vi "Test Production Unit API.vi"() -> ()   [LabVIEW 2025]
doc: "My Module API Tester.\n_____\nBased on DQMH Dev Tools: Project Template 7.1.2.1547."
uses:
  Production Unit.lvlib
  <vilib>/Utility/error.llb/DialogType.ctl
panel:
  out "last error":errorcluster
  in  "Show Diagram on Init":bool
  in  "Run as Singleton?":bool
  in  "Show Block Diagram":bool
  in  "Refresh Modules":bool
  out "Active Modules":string[](array[string])
  in  "Stop Module":bool
  in  "Select Module":i32(ring)=-1 caption="Select Module\nTo send Request to" items=["All"=-1]
  in  "Run New Module":bool
  in  "Hide Module Panel":bool
  in  "Show Module Panel":bool
  out "Status":string
  # "This VI tests the API for the Module."
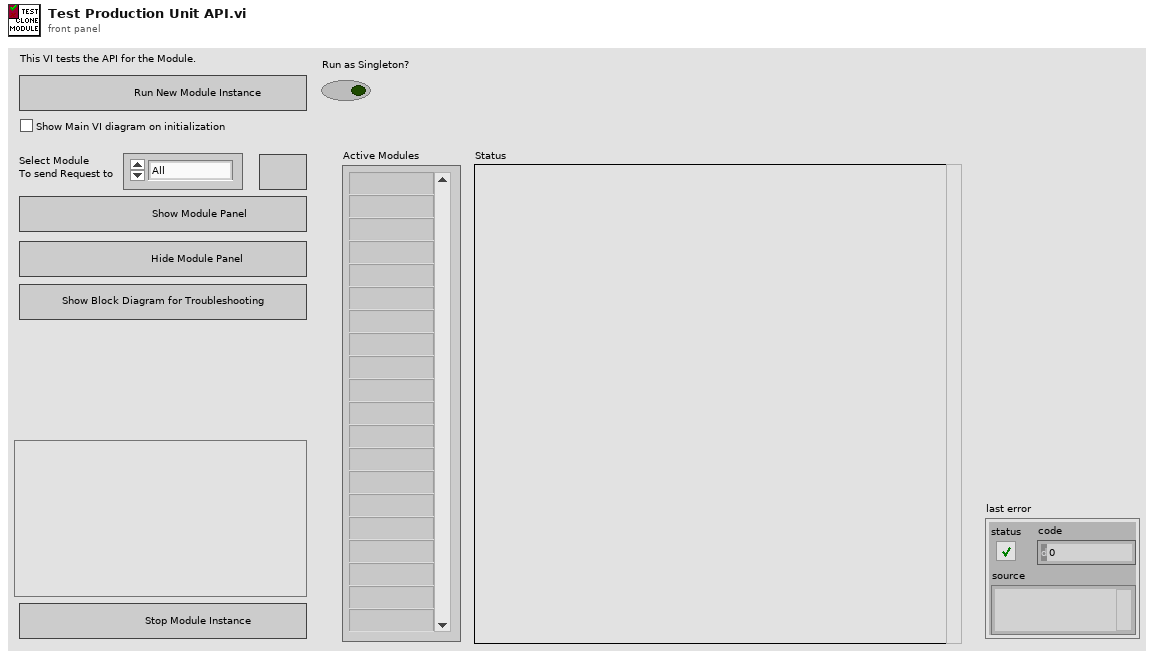
[diagram p1: front panel]
types:
  T1 = typedef "Production Unit.lvlib/Broadcast Events--cluster.ctl" = cluster{"Module Did Init":refnum<user-event>, "Status Updated":refnum<user-event>, "Error Reported":refnum<user-event>, "Module Did Stop":refnum<user-event>, "Update Module Execution Status":refnum<user-event>}
  T2 = typedef "DialogType.ctl" = u16
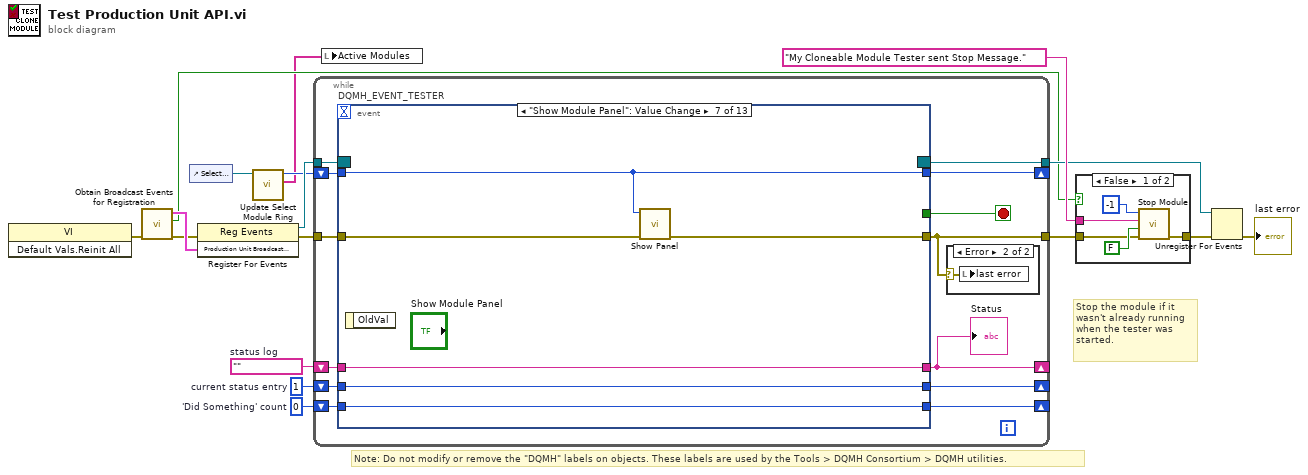
[diagram p0: block diagram]
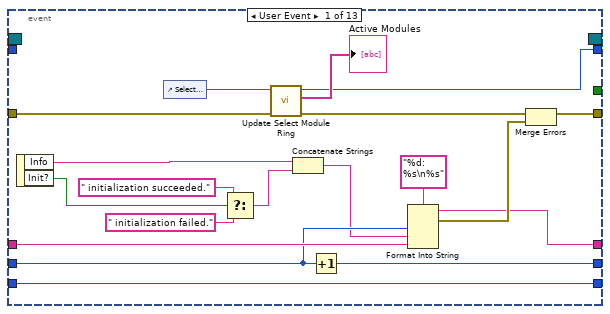
[diagram p4: hidden frame]
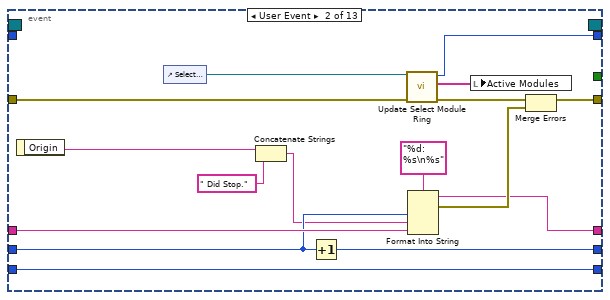
[diagram p5: hidden frame]
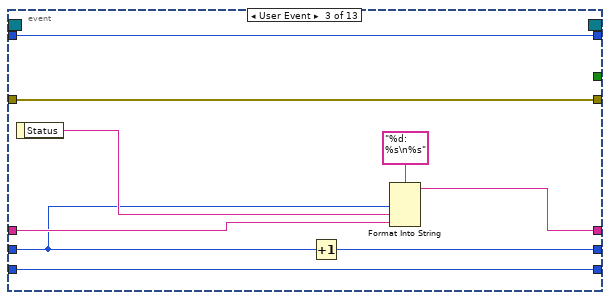
[diagram p6: hidden frame]
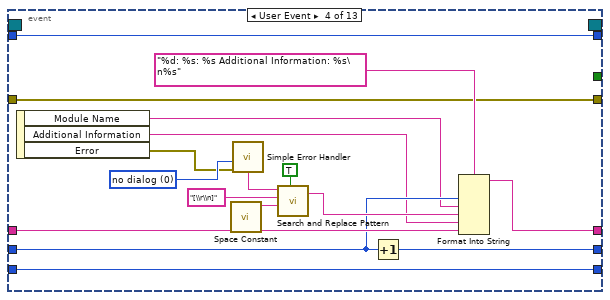
[diagram p7: hidden frame]
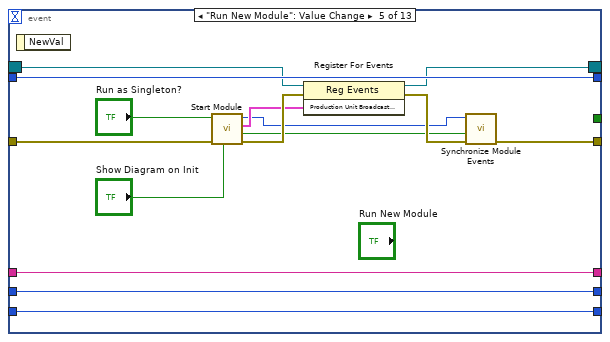
[diagram p8: hidden frame]
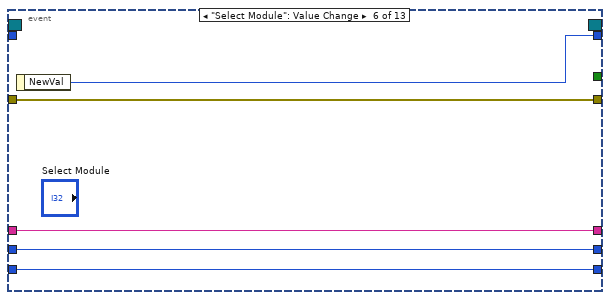
[diagram p9: hidden frame]
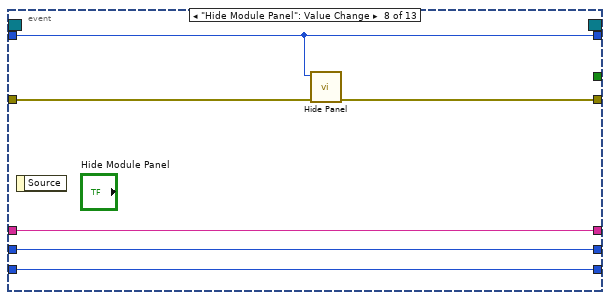
[diagram p10: hidden frame]
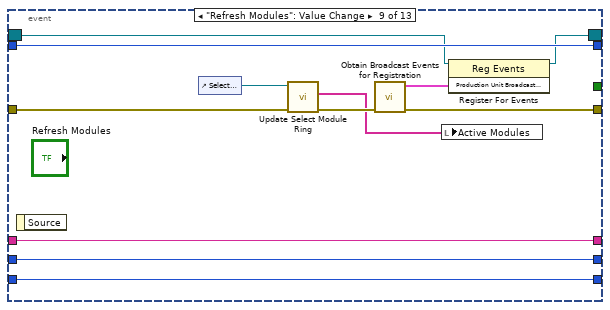
[diagram p11: hidden frame]
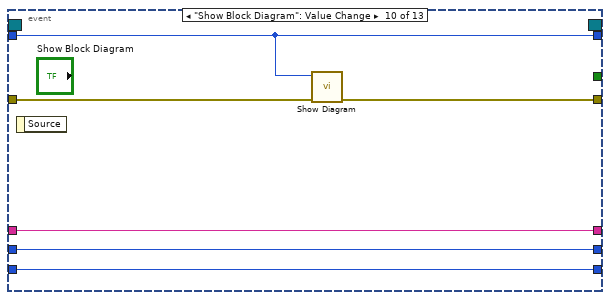
[diagram p12: hidden frame]
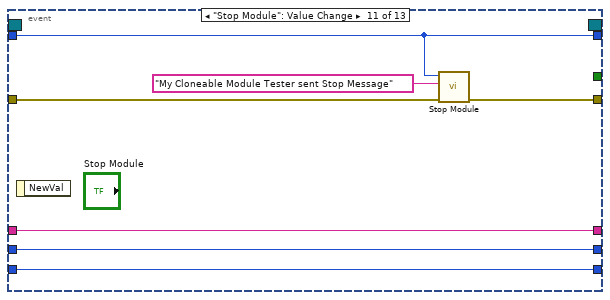
[diagram p13: hidden frame]
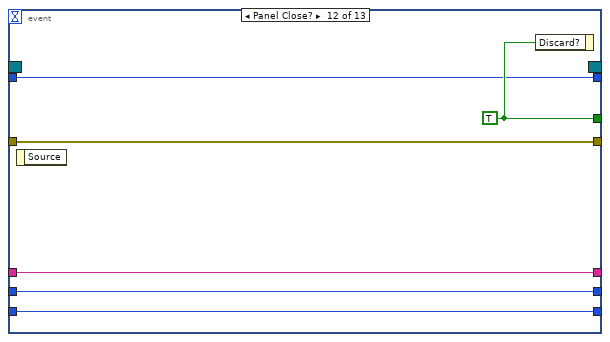
[diagram p14: hidden frame]
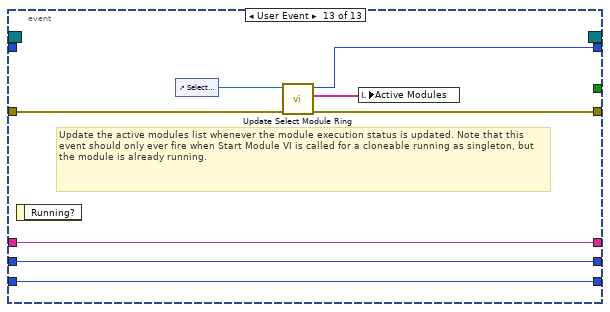
[diagram p15: hidden frame]
diagram:
  w13 = 0  # 'Did Something' count
  w14 = 1  # current status entry
  w15 = ""  # status log
  # "Stop the module if it wasn't already running when the tester was started."
  # "Note: Do not modify or remove the \"DQMH\" labels on objects. These labels are used by the Tools > DQMH Consortium > DQMH utilities."
  n1 = invoke class="VI" method="Default Vals.Reinit All"() -> (error out=w8:errorcluster)  [unwired: 3 in, 2 out]
  n2 = call "Obtain Broadcast Events for Registration.vi"("error in"=w8) -> ("error out"=w7:errorcluster, "Already running?"=w6:bool, "Production Unit Broadcast Events"=w12:T1)  [unwired: 8 in]
  n3 = control-ref of="Select Module"() -> (w3:refnum<vi>)
  n4 = register-events(error in=w7, w12) -> (reference out=w17:refnum<event-registration>, error out=w11:errorcluster)  [unwired: 1 in]
  n5 = call "Update Select Module Ring.vi"("Select Module Ring Ref"=w3) -> ("Active Modules (Array)"=w1:string[], "New Module Ring Value"=w2:i32)  [unwired: 8 in, 1 out]
  n6 = while {
    tunnel: w17 -> [w30]
    tunnel: [w19] -> w5
    tunnel: w11 -> [w29]
    shift-right: [w25] -> _
    shift-left: w15 -> [w27]
    shift-right: [w26] -> _
    shift-left: w14 -> [w28]
    shift-right: [w23] -> _
    shift-left: w13 -> [w24]
    shift-right: [w21] -> _
    shift-left: w2 -> [w22]
    tunnel: [w20] -> w9
    stop <- w18 stop-if-true
    n7 = event "DQMH_EVENT_TESTER" shown="[6] \"Show Module Panel\": Value Change" {
      selector: w30 -> [_ _ _ _ w100 _ _ _ w130 _ _ _ _]
      dyn-events: [_ _ _ _ w99 _ _ _ w129 _ _ _ _] -> w20
      timeout: _ -> [_ _ _ _ _ _ _ _ _ _ _ _ _]
      tunnel: [_ _ _ _ _ _ _ _ _ _ _ w155 _] -> w18
      tunnel: [w39 w57 w75 w79 w98 w112 w117 w123 w126 w138 w144 w154 w158] -> w19
      tunnel: w29 -> [w41 w59 w75 w79 w101 w112 w118 w124 w131 w142 w145 w154 w159]
      tunnel: w28 -> [w47 w63 w67 w82 w104 w110 w115 w121 w135 w140 w148 w152 w162]
      tunnel: w27 -> [w48 w64 w71 w83 w105 w111 w116 w122 w136 w141 w149 w153 w163]
      tunnel: [w45 w61 w72 w81 w105 w111 w116 w122 w136 w141 w149 w153 w163] -> w25
      tunnel: [w46 w62 w74 w80 w104 w110 w115 w121 w135 w140 w148 w152 w162] -> w26
      tunnel: w24 -> [w42 w60 w70 w92 w103 w109 w114 w120 w134 w139 w147 w151 w161]
      tunnel: [w42 w60 w70 w92 w103 w109 w114 w120 w134 w139 w147 w151 w161] -> w23
      tunnel: w22 -> [_ _ w68 w91 w102 _ w113 w119 w133 w137 w146 w150 _]
      tunnel: [w36 w54 w68 w91 w102 w108 w113 w119 w133 w137 w146 w150 w157] -> w21
      event User Event {
        n8 = event-data() -> ("Info"=w44:string, "Init?"=w33:bool)  [unwired: 1 in]
        n9 = control-ref of="Select Module"() -> (w38:refnum<vi>)
        n10 = Select(t=" initialization succeeded.", s=w33, f=" initialization failed.") -> (s? t:f=w32:string)
        n11 = call "Update Select Module Ring.vi"("error in"=w41, "Select Module Ring Ref"=w38) -> ("error out"=w40:errorcluster, "Active Modules (Array)"=→"Active Modules":string[], "New Module Ring Value"=w36:i32)  [unwired: 7 in]
        n12 = Concatenate Strings(w44, w32) -> (w43:string)
        n13 = Increment(x=w47) -> (x+1=w46:i32)
        n14 = Format Into String(format string="%d: %s\n%s", w47, w43, w48) -> (resulting string=w45:string, error out=w50:errorcluster)  [unwired: 2 in]
        n15 = Merge Errors(w40, w50) -> (w39:errorcluster)
      }
      event User Event {
        n16 = event-data() -> ("Origin"=w52:string)  [unwired: 1 in]
        n17 = control-ref of="Select Module"() -> (w56:refnum<vi>)
        n18 = Concatenate Strings(w52, " Did Stop.") -> (w51:string)
        n19 = Increment(x=w63) -> (x+1=w62:i32)
        n20 = call "Update Select Module Ring.vi"("error in"=w59, "Select Module Ring Ref"=w56) -> ("error out"=w58:errorcluster, "Active Modules (Array)"=w55:string[], "New Module Ring Value"=w54:i32)  [unwired: 7 in]
        n21 = Format Into String(format string="%d: %s\n%s", w63, w51, w64) -> (resulting string=w61:string, error out=w66:errorcluster)  [unwired: 2 in]
        n22 = local write "Active Modules"(w55) -> ()
        n23 = Merge Errors(w58, w66) -> (w57:errorcluster)
      }
      event User Event {
        n24 = event-data() -> ("Status"=w69:string)  [unwired: 1 in]
        n25 = Increment(x=w67) -> (x+1=w74:i32)
        n26 = Format Into String(format string="%d: %s\n%s", w67, w69, w71) -> (resulting string=w72:string)  [unwired: 2 in, 1 out]
      }
      event User Event {
        w84 = T2 0 items=["no dialog", "OK message", "continue or stop message", "OK message + warnings", "continue/stop + warnings"] ("type of dialog (OK msg:1)")
        n27 = event-data() -> ("Module Name"=w78:string, "Additional Information"=w77:string, "Error"=w76:errorcluster)  [unwired: 1 in]
        n28 = call <vilib>:"Space Constant.vi"() -> ("String"=w88:string)
        n29 = call <vilib>:"Simple Error Handler.vi"("type of dialog (OK msg:1)"=w84, "error in (no error)"=w76) -> ("message"=w85:string)  [unwired: 3 in, 4 out]
        n30 = call <vilib>:"Search and Replace Pattern.vi"("string"=w85, "regular expression (\"\")"="[\\r\\n]" ("regular expression (\"\")"), "replace string (\"\")"=w88, "replace all? (F)"=TRUE ("replace all CR/LF with spaces")) -> ("result string"=w86:string)  [unwired: 1 in, 1 out]
        n31 = Increment(x=w82) -> (x+1=w80:i32)
        n32 = Format Into String(format string="%d: %s: %s Additional Information: %s\n%s", w82, w78, w86, w77, w83) -> (resulting string=w81:string)  [unwired: 2 in, 1 out]
      }
      event "Run New Module": Value Change {
        n33 = event-data() -> ()  [unwired: 1 in, 1 out]
        n34 = call "Start Module.vi"("Show Main VI Diagram on Init (F)"="Show Diagram on Init", "error in"=w101, "Run as Singleton? (F)"="Run as Singleton?") -> ("error out"=w106:errorcluster, "Wait for Event Sync?"=w97:bool, "Production Unit Broadcast Events"=w96:T1, "Module ID"=w93:i32)  [unwired: 4 in, 1 out]
        n35 = register-events(reference=w100, error in=w106, w96) -> (reference out=w99:refnum<event-registration>, error out=w107:errorcluster)
        n36 = call "Synchronize Module Events.vi"("error in"=w107, "Wait for Event Sync?"=w97, "Module ID in"=w93) -> ("error out"=w98:errorcluster)  [unwired: 7 in, 1 out]
      }
      event "Select Module": Value Change {
        n37 = event-data() -> ("NewVal"=w108:i32)  [unwired: 1 in]
      }
      event "Show Module Panel": Value Change {
        n38 = event-data() -> ()  [unwired: 1 in, 1 out]
        n39 = call "Show Panel.vi"("error in"=w118, "Module ID"=w113) -> ("error out"=w117:errorcluster)  [unwired: 9 in]
      }
      event "Hide Module Panel": Value Change {
        n40 = event-data() -> ()  [unwired: 1 in, 1 out]
        n41 = call "Hide Panel.vi"("error in"=w124, "Module ID"=w119) -> ("error out"=w123:errorcluster)  [unwired: 9 in]
      }
      event "Refresh Modules": Value Change {
        n42 = event-data() -> ()  [unwired: 1 in, 1 out]
        n43 = control-ref of="Select Module"() -> (w132:refnum<vi>)
        n44 = call "Update Select Module Ring.vi"("error in"=w131, "Select Module Ring Ref"=w132) -> ("error out"=w127:errorcluster, "Active Modules (Array)"=w125:string[])  [unwired: 7 in, 1 out]
        n45 = call "Obtain Broadcast Events for Registration.vi"("error in"=w127) -> ("error out"=w126:errorcluster, "Production Unit Broadcast Events"=w128:T1)  [unwired: 8 in, 1 out]
        n46 = local write "Active Modules"(w125) -> ()
        n47 = register-events(reference=w130, w128) -> (reference out=w129:refnum<event-registration>)  [unwired: 1 in, 1 out]
      }
      event "Show Block Diagram": Value Change {
        n48 = event-data() -> ()  [unwired: 1 in, 1 out]
        n49 = call "Show Diagram.vi"("error in"=w142, "Module ID"=w137) -> ("error out"=w138:errorcluster)  [unwired: 9 in]
      }
      event "Stop Module": Value Change {
        n50 = event-data() -> ()  [unwired: 1 in, 1 out]
        n51 = call "Stop Module.vi"("error in"=w145, "Origin"="My Cloneable Module Tester sent Stop Message", "Module ID"=w146) -> ("error out"=w144:errorcluster)  [unwired: 8 in]
      }
      event Panel Close? {
        w155 = TRUE ("Discard?")
        n52 = event-data() -> ()  [unwired: 1 in, 1 out]
        n53 = event-data("Discard?"=w155) -> ()  [unwired: 1 in, 1 out]
      }
      event User Event {
        # "Update the active modules list whenever the module execution status is updated. Note that this event should only ever fire when Start Module VI is called for a cloneable running as singleton, but the module is already running."
        n54 = event-data() -> ()  [unwired: 1 in, 1 out]
        n55 = control-ref of="Select Module"() -> (w160:refnum<vi>)
        n56 = call "Update Select Module Ring.vi"("error in"=w159, "Select Module Ring Ref"=w160) -> ("error out"=w158:errorcluster, "Active Modules (Array)"=w156:string[], "New Module Ring Value"=w157:i32)  [unwired: 7 in]
        n57 = local write "Active Modules"(w156) -> ()
      }
    }
    "Status" <- w25
    n58 = case shown="Error" w19 {
      selector: w19 -> [_ w31]
      frame No Error {
      }
      frame Error {
        n59 = local write "last error"(w31) -> ()
      }
    }
  }
  n60 = local write "Active Modules"(w1) -> ()
  n61 = case shown="False" w6 {
    tunnel: [w168 w169] -> w16
    tunnel: "My Cloneable Module Tester sent Stop Message." ("Origin") -> [w167 _]
    tunnel: w5 -> [w164 w169]
    frame False {
      n62 = call "Stop Module.vi"("error in"=w164, "Wait for Module to stop? (F)"=FALSE ("Wait for Module to stop?"), "Origin"=w167, "Module ID"=-1 ("Stop all")) -> ("error out"=w168:errorcluster)  [unwired: 7 in]
    }
    frame True {
    }
  }
  n63 = Unregister For Events(event registration refnum=w9, error in=w16) -> (error out=→"last error":errorcluster)
